vi "Initialize_Robcomm.vi"(0 "working directory":path=path "C:/RCWIN", 1 "command line":string="C:\\RCWIN\\Robot.exe") -> (2 "return code":i32, 3 "DDE Service name":string="ROBCOMM", 4 "error out":errorcluster)   [LabVIEW 2012]
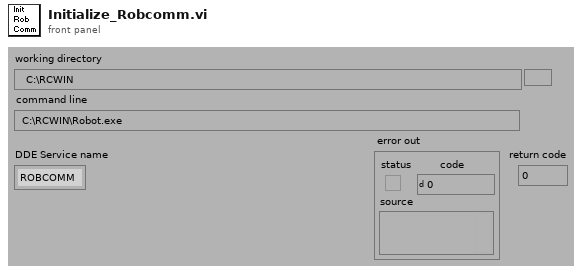
[diagram p1: front panel]
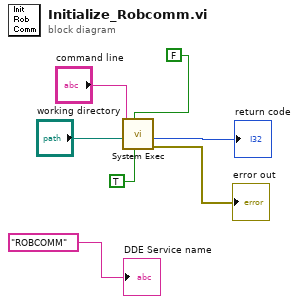
[diagram p0: block diagram]
diagram:
  n1 = call <vilib>:"System Exec.vi"("run minimized? (F)"=TRUE, "wait until completion? (T)"=FALSE, "working directory"="working directory", "command line"="command line") -> ("error out"=→"error out":errorcluster, "return code"=→"return code":i32)  [unwired: 4 in, 2 out]
  "DDE Service name" <- "ROBCOMM" ("DDE Service name")
